vi "DAQProducer.vi"(2 "Min Sample Rate":dbl=500000.0 format="%.2p", 3 "# Channels":i32=7, 4 "Samples Per Fetch":i32, 5 "Data Queue":refnum<queue>) -> (0 "error out":errorcluster)   [LabVIEW 2012]
uses:
  <instrlib>/niScope/Configure/Trigger/niScope Configure Trigger Software.vi
  ExecutionControlGlobal.vi
  <instrlib>/niScope/Acquire/Fetch/niScope Multi Fetch.vi
panel:
  out "Input Impedance":dbl=4.0 format="%.2f"
  out "Data Transfer Rate (MB/s)":dbl format="%.3p"
  out "Channel\nNumbers":string="0:6"
  out "actual sample rate":dbl caption="Actual Sample Rate" format="%.3p"
  in  "vertical range":dbl=5.0 format="%.2f"
  out "Total Samples Fetched":u64 format="%.3p"
  out "Total Acquired Data (bytes)":u64 format="%.3p"
  out "Time Delta":dbl
  out "Samples Used in Onboard Memory":i32(slide)=3898016 scale=-1.0..9586980.57142857 scale format="%.1p"
  in  "Total Duration of Acquisition (s)":u64=100000000 step=1048576 format="%.3p"
  out "Total Samples to Acquire":u64=100000000 step=1048576 format="%.3p"
  in  "Resource Name":refnum<k15>="Dev1"
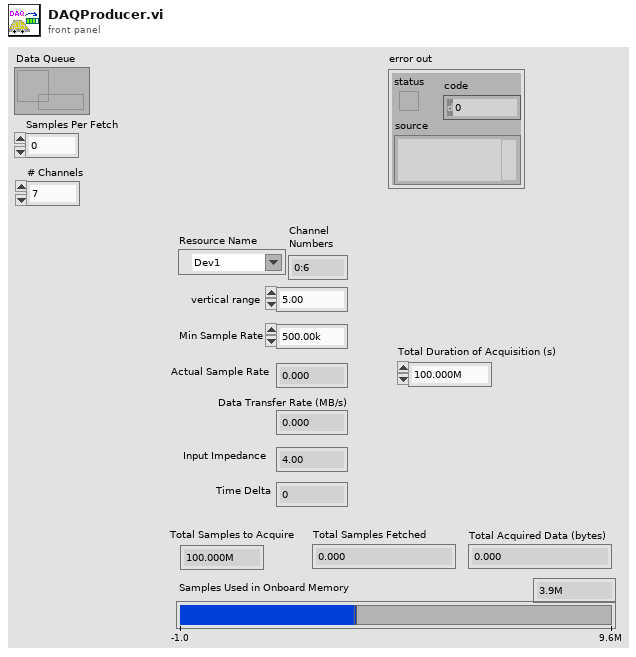
[diagram p1: front panel]
types:
  T1 = cluster{"actualSamples":i32, "absoluteInitialX":dbl, "relativeInitialX":dbl, "xIncrement":dbl, "offset":dbl, "gain":dbl, "reserved1":dbl, "reserved2":dbl}[]
  T2 = cluster{"actualSamples":i32, "absoluteInitialX":dbl, "relativeInitialX":dbl, "xIncrement":dbl, "offset":dbl, "gain":dbl, "reserved1":dbl, "reserved2":dbl}
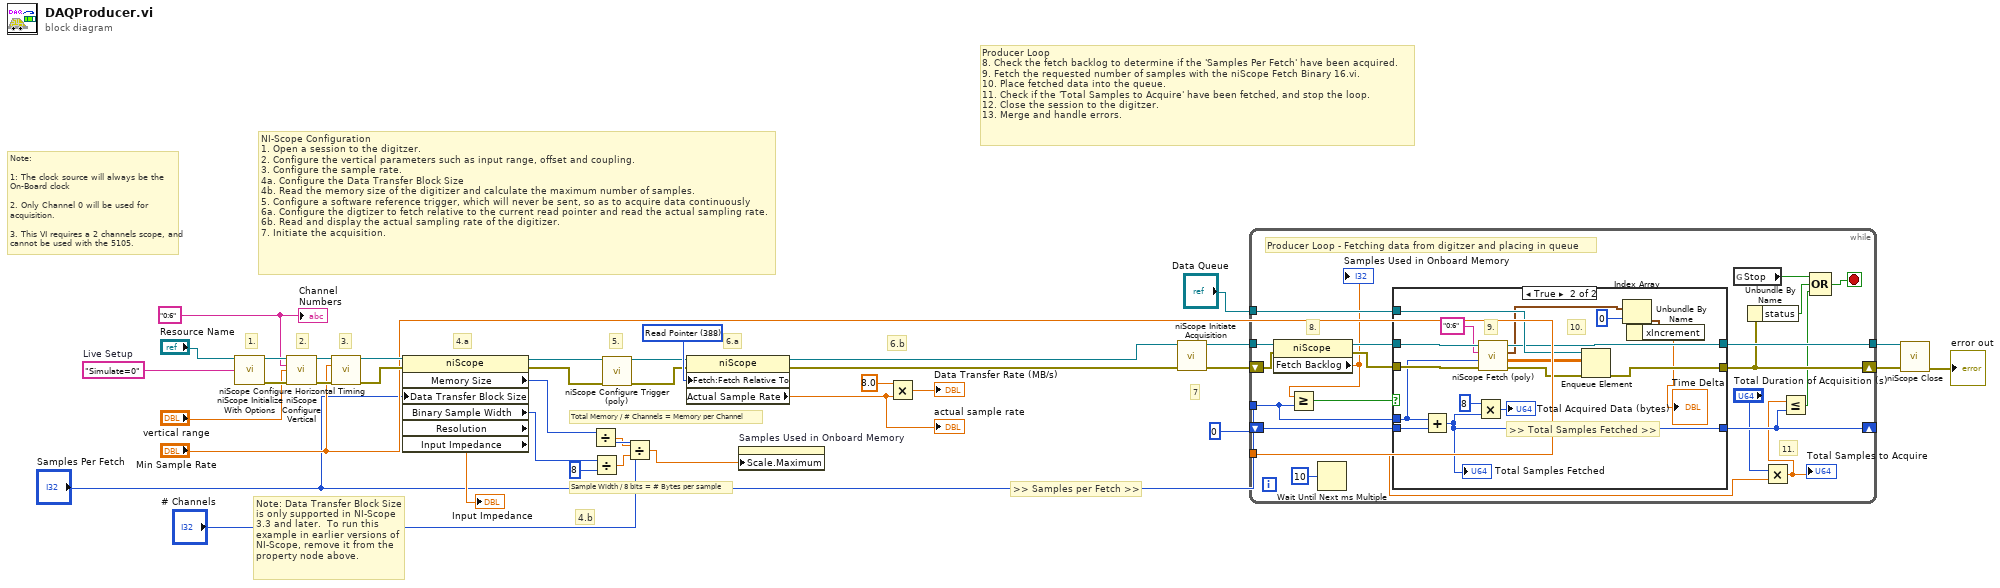
[diagram p0: block diagram]
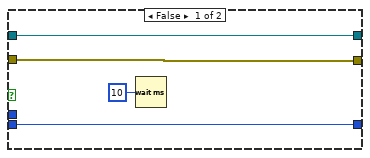
[diagram p2: hidden frame]
diagram:
  w9 = "Simulate=0"  # Live Setup
  w16 = "0:6"
  w31 = 388 items=["Start"=482, "Trigger"=483, "Pretrigger"=477, "Now"=481, "Read Pointer"=388] ("Fetch:Fetch Relative To")
  # ">> Samples per Fetch >>"
  # "Total Memory / # Channels = Memory per Channel"
  # "Sample Width / 8 bits = # Bytes per sample"
  # "Note: \n\n1: The clock source will always be the \nOn-Board clock\n\n2. Only Channel 0 will be used for acquisition.\n\n3. This VI requires a 2 channels scope, and \ncannot be used with the 5105."
  # "Note: Data Transfer Block Size is only supported in NI-Scope 3.3 and later.  To run this example in earlier versions of NI-Scope, remove it from the property node above."
  # "Producer Loop\n8. Check the fetch backlog to determine if the 'Samples Per Fetch' have been acquired.\n9. Fetch the requested number of samples with the niScope Fetch Binary 16.vi.\n10. Place fetched data into the queue.\n11. Check if the 'Total Samples to Acquire' have been fetched, and stop the loop.\n12. Close the session to the digitzer.\n13. Merge and handle errors."
  # "6.b"
  # "7"
  # "6.a"
  # "5."
  # "4.b"
  # "4.a"
  # "3."
  # "2."
  # "1."
  # "NI-Scope Configuration\n1. Open a session to the digitzer.\n2. Configure the vertical parameters such as input range, offset and coupling.\n3. Configure the sample rate.\n4a. Configure the Data Transfer Block Size\n4b. Read the memory size of the digitizer and calculate the maximum number of samples.\n5. Configure a software reference trigger, which will never be sent, so as to acquire data continuously\n6a. Configure the digtizer to fetch relative to the current read pointer and read the actual sampling rate.\n6b. Read and display the actual sampling rate of the digitizer.\n7. Initiate the acquisition."
  n1 = call <instrlib>:"niScope Initialize With Options.vi"("resource name"="Resource Name", "option string"=w9) -> ("instrument handle"=w36:refnum<k15>, "error out"=w35:errorcluster)  [unwired: 12 in]
  n2 = call <instrlib>:"niScope Configure Vertical.vi"("instrument handle"=w36, "channels"=w16, "vertical range"="vertical range", "error in"=w35) -> ("instrument handle out"=w34:refnum<k15>, "error out"=w33:errorcluster)  [unwired: 10 in]
  n3 = call <instrlib>:"niScope Configure Horizontal Timing.vi"("instrument handle"=w34, "min sample rate"="Min Sample Rate", "error in"=w33) -> ("instrument handle out"=w22:refnum<k15>, "error out"=w26:errorcluster)  [unwired: 11 in]
  n4 = property class="niScope" props=["Memory Size", "Data Transfer Block Size", "Binary Sample Width", "Resolution", "Input Impedance"](reference=w22, error in=w26, "Data Transfer Block Size"="Samples Per Fetch") -> (reference out=w23:refnum<k15>, error out=w25:errorcluster, "Memory Size"=w24:i32, "Binary Sample Width"=w19:i32, "Input Impedance"=→"Input Impedance":dbl)  [unwired: 1 out]
  n5 = Divide(x=w24, y="# Channels") -> (x/y=w15:dbl)
  n6 = Divide(x=w19, y=8) -> (x/y=w14:dbl)
  n7 = call-poly <instrlib>:"niScope Configure Trigger (poly).vi"("instrument handle"=w23, "error in"=w25) -> ("instrument handle out"=w30:refnum<k15>, "error out"=w29:errorcluster)  [unwired: 12 in]
  n8 = Divide(x=w15, y=w14) -> (x/y=w6:dbl)
  n9 = property class="niScope"(reference=w30, error in=w29, "Fetch:Fetch Relative To"=w31) -> (reference out=w17:refnum<k15>, error out=w8:errorcluster, "Actual Sample Rate"=w12:dbl)
  "actual sample rate" <- w12
  n10 = property on="Samples Used in Onboard Memory" class="Slide (strict)"("Scale.Maximum"=w6) -> ()  [unwired: 2 in, 2 out]
  n11 = Multiply(x=8.0, y=w12) -> (x*y=→"Data Transfer Rate (MB/s)":dbl)
  n12 = call <instrlib>:"niScope Initiate Acquisition.vi"("instrument handle"=w17, "error in"=w8) -> ("instrument handle out"=w28:refnum<k15>, "error out"=w27:errorcluster)  [unwired: 12 in]
  n13 = while {
    tunnel: w28 -> [w49]
    tunnel: [w57] -> w2
    shift-right: [w45] -> _
    shift-left: u64 0 ("Samples to Take") -> [w46]
    tunnel: "Data Queue" -> [w52]
    shift-right: [w56] -> w4
    shift-left: w27 -> [w51]
    tunnel: "Samples Per Fetch" -> [w47]
    tunnel: "Min Sample Rate" -> [w41]
    stop <- w54 stop-if-true
    # "11."
    # "8."
    # "Producer Loop - Fetching data from digitzer and placing in queue"
    n14 = property class="niScope"(reference=w49, error in=w51) -> (reference out=w48:refnum<k15>, error out=w50:errorcluster, "Fetch Backlog"=w44:dbl)
    "Samples Used in Onboard Memory" <- w44
    n15 = Greater Or Equal?(x=w44, y=w47) -> (x >= y?=w39:bool)
    n16 = Wait Until Next ms Multiple(millisecond multiple=u32 10) -> ()  [unwired: 1 out]
    n17 = case shown="True" w39 {
      tunnel: [w61 w67] -> w57
      tunnel: [w60 w68] -> w56
      tunnel: w52 -> [_ w77]
      tunnel: w50 -> [w60 w76]
      tunnel: w48 -> [w61 w75]
      tunnel: w47 -> [_ w70]
      tunnel: w46 -> [w59 w74]
      tunnel: [w59 w73] -> w45
      frame False {
        n18 = Wait (ms)(milliseconds to wait=u32 10) -> ()  [unwired: 1 out]
      }
      frame True {
        # ">> Total Samples Fetched >>"
        # "10."
        # "9."
        n19 = Add(x=w70, y=w74) -> (x+y=w73:u64)
        "Total Samples Fetched" <- w73
        n20 = Multiply(x=u64 8, y=w73) -> (x*y=→"Total Acquired Data (bytes)":u64)
        n21 = call-poly <instrlib>:"niScope Fetch (poly).vi"("error in"=w76, "numSamples"=w70, "channels"="0:6" ("channel"), "instrument handle"=w75) -> ("error out"=w78:errorcluster, "wfm"=w62:dbl[][], "wfm info"=w65:T1, "instrument handle out"=w67:refnum<k15>)  [unwired: 4 in]
        n22 = Enqueue Element(queue=w77, element=w62, error in (no error)=w78) -> (error out=w68:errorcluster)  [unwired: 1 in, 2 out]
        n23 = Index Array(array=w65, index=0) -> (element=w64:T2)
        n24 = Unbundle By Name(w64) -> ("xIncrement"=→"Time Delta":dbl)
      }
    }
    n25 = global read "ExecutionControlGlobal.vi" "Stop"() -> (w38:bool)
    n26 = Unbundle By Name(w56) -> ("status"=w55:bool)
    n27 = Multiply(x="Total Duration of Acquisition (s)", y=w41) -> (x*y=w40:dbl)
    "Total Samples to Acquire" <- w40
    n28 = Less Or Equal?(x=w40, y=w45) -> (x <= y?=w53:bool)
    n29 = Compound Arithmetic op=OR(w38, w55, w53) -> (w54:bool)
  }
  n30 = call <instrlib>:"niScope Close.vi"("instrument handle"=w2, "error in"=w4) -> ("error out"=→"error out":errorcluster)  [unwired: 13 in]
  "Channel\nNumbers" <- w16
